vi "dfd_Validate Params for Comb Design by N.vi"(6 "fs [Hz]":dbl=1.0 format="%.2f", 8 "error in (no error)":errorcluster, 9 "bandwidth [Hz]":dbl=0.2 format="%.2f", 10 "Ab [dB]":dbl=3.010299956639812 format="%#.6g", 11 "order":i32) -> (0 "error out":errorcluster, 1 "normalized BW [rad/s]":dbl format="%.2f", 2 "dup Ab [dB]":dbl format="%.2f", 3 "dup order":i32)   [LabVIEW 2017, in "NI_DigFilter_Design.lvlib"]
uses:
  <vilib>/addons/Digital Filter Design/NI_DigFilter_Design.lvlib
  <vilib>/addons/Digital Filter Design/_Misc.llb/dfd_Error Handlers (Multiple).vi
  <vilib>/addons/Digital Filter Design/NI_DigFilterLicensed.lvlib
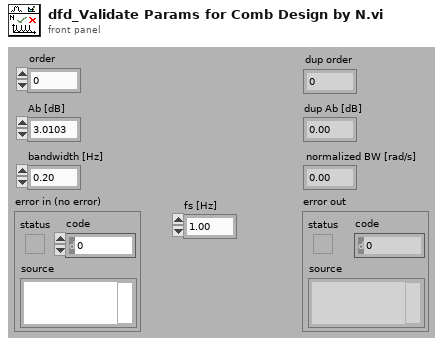
[diagram p1: front panel]
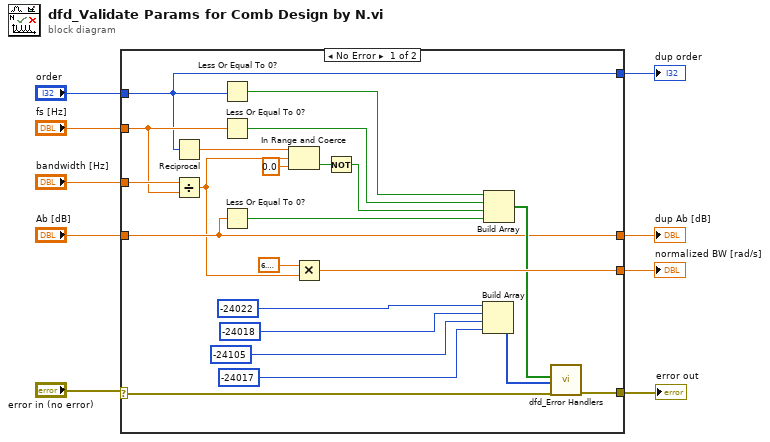
[diagram p0: block diagram]
diagram:
  n1 = case shown="No Error" "error in (no error)" {
    selector: "error in (no error)" -> [w27 w32]
    tunnel: [w26 _] -> w9
    tunnel: "Ab [dB]" -> [w26 _]
    tunnel: "bandwidth [Hz]" -> [w22 _]
    tunnel: [w31 _] -> w6
    tunnel: "order" -> [w10 _]
    tunnel: [w30 w32] -> w5
    tunnel: [w10 _] -> w2
    tunnel: "fs [Hz]" -> [w21 _]
    frame No Error {
      n2 = Reciprocal(x=w10) -> (1/x=w14:dbl)
      n3 = Divide(x=w22, y=w21) -> (x/y=w15:dbl)
      n4 = Less Or Equal To 0?(x=w10) -> (x <= 0?=w16:bool)
      n5 = Less Or Equal To 0?(x=w21) -> (x <= 0?=w23:bool)
      n6 = Less Or Equal To 0?(x=w26) -> (x <= 0?=w24:bool)
      n7 = In Range and Coerce(upper limit=w14, x=w15, lower limit=0.0) -> (In Range?=w12:bool)  [unwired: 1 out]
      n8 = Multiply(x=6.283185307179586, y=w15) -> (x*y=w31:dbl)
      n9 = Not(x=w12) -> (.not. x?=w11:bool)
      n10 = Build Array(-24022 ("ERR_ORDER_LE_ZERO"), -24018 ("ERR_FS_LE_ZERO"), -24105 ("ERR_COMB_BW_BYN_RANGE_WRONG"), -24017 ("ERR_dB_LE_ZERO")) -> (w28:i32[])
      n11 = Build Array(w16, w23, w11, w24) -> (w29:bool[])
      n12 = call-poly <vilib>:"dfd_Error Handlers.vi"("error in (no error)"=w27, "error sources"=w28, "condition failed?"=w29) -> ("error out"=w30:errorcluster)  [unwired: 8 out]
    }
    frame Error {
    }
  }
  "dup Ab [dB]" <- w9
  "normalized BW [rad/s]" <- w6
  "error out" <- w5
  "dup order" <- w2
